vi "Global Drive Variables.vi"() -> ()   [LabVIEW 2015]
uses:
  JoystickData.ctl
panel:
  out "Joystick Data":T1
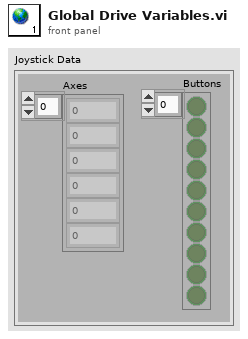
[diagram p1: front panel]
types:
  T1 = typedef "JoystickData.ctl" = cluster{"Axes":dbl[], "Buttons":bool[]}
diagram:
